vi "Action.vi"(8 "error in (no error)":errorcluster, 10 "Actor in":refnum<class "Tamagotchi Basic Actor.lvclass">, 11 "Update Cycles Message in":refnum<class "Update Cycles Message.lvclass">) -> (0 "error out":errorcluster, 2 "Actor out":refnum<class "Tamagotchi Basic Actor.lvclass">, 3 "Update Cycles Message out":refnum<class "Update Cycles Message.lvclass">)   [LabVIEW 2026, in "Update Cycles Message.lvclass"]
uses:
  Update Cycles Message.lvclass
  Tamagotchi Basic Actor/Tamagotchi Basic Actor.lvclass
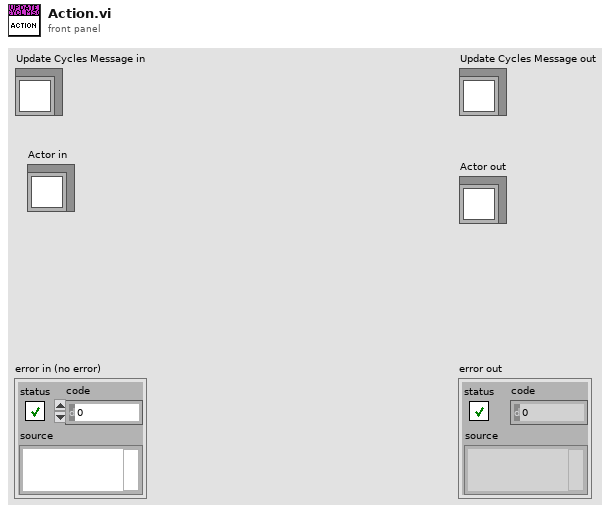
[diagram p1: front panel]
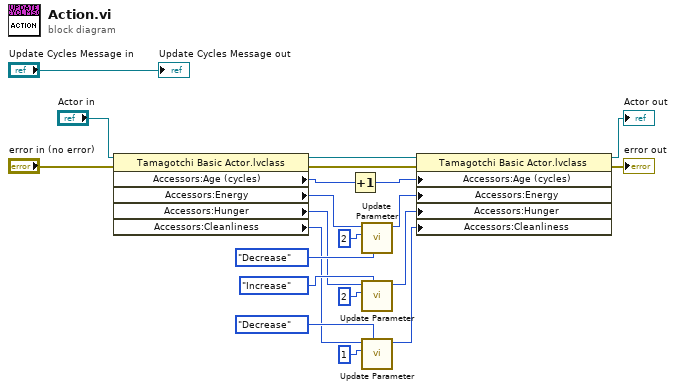
[diagram p0: block diagram]
diagram:
  n1 = property class="Tamagotchi Basic Actor.lvclass"(reference="Actor in", error in="error in (no error)") -> (reference out=w19:refnum<class "Tamagotchi Basic Actor.lvclass">, error out=w1:errorcluster, "Accessors:Age (cycles)"=w11:u32, "Accessors:Energy"=w10:i16, "Accessors:Hunger"=w9:i16, "Accessors:Cleanliness"=w8:i16)
  n2 = Increment(x=w11) -> (x+1=w7:u32)
  n3 = call "Update Parameter.vi"("Action"=enum16{"Increase", "Decrease"}."Decrease", "Modifier"=i16 2, "Parameter"=w10) -> ("New Value"=w6:i16)  [unwired: 8 in]
  n4 = call "Update Parameter.vi"("Action"=enum16{"Increase", "Decrease"}."Increase", "Modifier"=i16 2, "Parameter"=w9) -> ("New Value"=w5:i16)  [unwired: 8 in]
  n5 = call "Update Parameter.vi"("Action"=enum16{"Increase", "Decrease"}."Decrease", "Modifier"=i16 1, "Parameter"=w8) -> ("New Value"=w4:i16)  [unwired: 8 in]
  n6 = property class="Tamagotchi Basic Actor.lvclass"(reference=w19, error in=w1, "Accessors:Age (cycles)"=w7, "Accessors:Energy"=w6, "Accessors:Hunger"=w5, "Accessors:Cleanliness"=w4) -> (reference out=→"Actor out":refnum<class "Tamagotchi Basic Actor.lvclass">, error out=→"error out":errorcluster)
  "Update Cycles Message out" <- "Update Cycles Message in"
